vi "Get Instr Identifier.vi"(8 "error in (no error)":errorcluster, 11 "Configuration Base in":refnum<class "CFG Base.lvclass">) -> (0 "error out":errorcluster, 2 "Instr Identifier":string, 3 "Configuration Base out":refnum<class "CFG Base.lvclass">)   [LabVIEW 2023, in "HAL GOOP4.lvlib" / "CFG Base.lvclass"]
uses:
  CFG Base.lvclass
  93c41ed1-0e68-4773-967c-815ca95f02ed.vi
  <vilib>/ErrorRing/Error Ring.xnode
  <vilib>/Utility/error.llb/Error Cluster From Error Code.vi
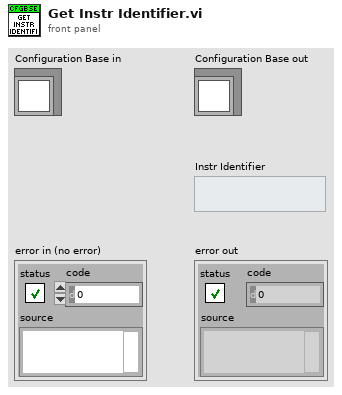
[diagram p1: front panel]
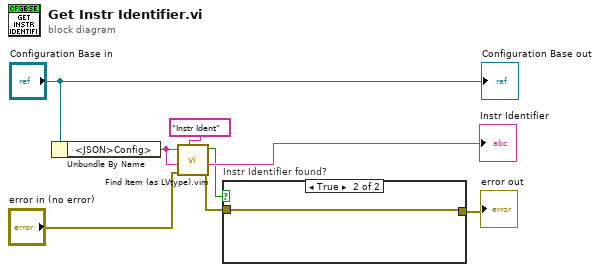
[diagram p0: block diagram]
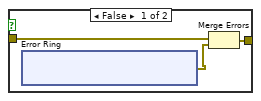
[diagram p2: hidden frame]
diagram:
  n1 = Unbundle By Name("Configuration Base in") -> ("<JSON>Config>"=w5:string)
  n2 = call "Find Item (as LVtype).vim"("$Path or Item Name"="Instr Ident", "error in (no error)"="error in (no error)", "Data Type and Default Value"=w5, "JSON"=w5) -> ("error out"=w2:errorcluster, "Data"=→"Instr Identifier":string, "Found"=w3:bool)  [unwired: 4 in, 1 out]
  n3 = case "Instr Identifier found?" shown="True" w3 {
    tunnel: w2 -> [w10 w17]
    tunnel: [w9 w17] -> w1
    frame False {
      n4 = xnode "Error Ring"() -> ("error out"=w11:errorcluster)
      n5 = Merge Errors(w10, w11) -> (w9:errorcluster)
    }
    frame True {
    }
  }
  "error out" <- w1
  "Configuration Base out" <- "Configuration Base in"
